vi "dvl sim (SubVI).vi"(0 "IC_Water_depth":dbl=50.0, 1 "a2":dbl, 2 "b2":dbl, 5 "a1":dbl=-0.1, 9 "b1":dbl=0.2, 13 "eta":dbl[](array[numeric])) -> (3 "f_xy":dbl, 4 "dvl_1":dbl, 6 "dvl_2":dbl, 8 "alt":dbl, 10 "dvl_3":dbl, 14 "DVL_alts":dbl[](array[numeric]), 15 "dvl_4":dbl)   [LabVIEW 2014]
uses:
  <vilib>/imath/engines/lvmath2/RunTimeEngine/IndexRead/NIMS V(S).vi
  <instcachedir>/0/NIMS V(S)_0488751826AF41519A22953C041130DC.lvgen/NIMS V(S)_0488751826AF41519A22953C041130DC_000.vi
  <vilib>/imathl/engines/lvmath/Functions/Error Handling/Create Error.vi
  <vilib>/imath/engines/lvmath2/RunTimeEngine/ArithmeticOperatorToken/NIMS_ArithmeticOperator_multmx(M,CV)-internal.vi
  <instcachedir>/0/NIMS_ArithmeticOperator_multmx(M,CV)-internal_25C7CE5937BA4322B5BE2717374345EA.lvgen/NIMS_ArithmeticOperator_multmx(M,CV)-internal_25C7CE5937BA4322B5BE2717374345EA_001.vi
  <vilib>/imath/engines/lvmath2/RunTimeEngine/RangeToken/NIMS_Range_R2 - Integer.vi
  <instcachedir>/0/NIMS_Range_R2 - Integer_2D1304BAF97744E0A293025746CBADFC.lvgen/NIMS_Range_R2 - Integer_2D1304BAF97744E0A293025746CBADFC_000.vi
  <vilib>/imath/engines/lvmath2/RunTimeEngine/CommandStatement/MC_CommandStatement_break.vi
  <vilib>/imath/engines/lvmath2/RunTimeEngine/ErrorHandling/NIMS_Create Error From Enums.vi
  <instcachedir>/0/NIMS V(S)_0488751826AF41519A22953C041130DC.lvgen/NIMS V(S)_0488751826AF41519A22953C041130DC_008.vi
  <vilib>/imath/engines/lvmath2/RunTimeEngine/IndexReplace/NIMS V(S)=S.vi
  <instcachedir>/0/NIMS V(S)=S_2D52C4EC15D8415E870AEE69FB516CCA.lvgen/NIMS V(S)=S_2D52C4EC15D8415E870AEE69FB516CCA_001.vi
  <instcachedir>/0/NIMS V(S)_0488751826AF41519A22953C041130DC.lvgen/NIMS V(S)_0488751826AF41519A22953C041130DC_006.vi
  <vilib>/imath/engines/lvmath2/RunTimeEngine/NodeEndStatement/NIMS_NodeEndStatement_Output.vi
  <instcachedir>/0/NIMS_NodeEndStatement_Output_53EC0D466D134D7ABD903AC30B43404B.lvgen/NIMS_NodeEndStatement_Output_53EC0D466D134D7ABD903AC30B43404B_001.vi
  <vilib>/imath/engines/lvmath2/RunTimeEngine/ErrorHandling/NIMS_Finalize Error.vi
panel:
  in  "dvl_do":i8[](array[numeric])=[1, 1, 1, 1]
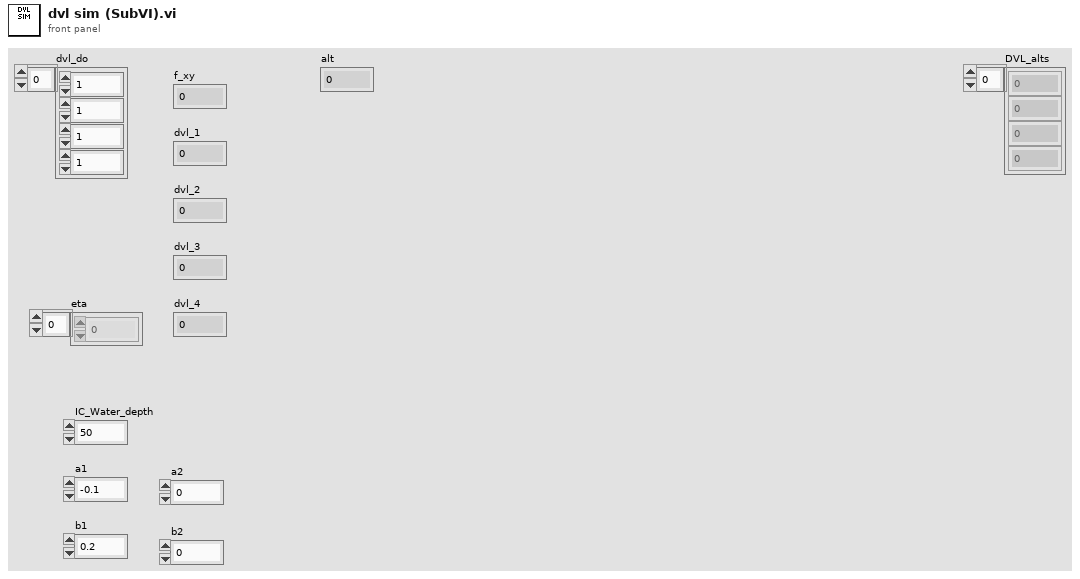
[diagram p1: front panel]
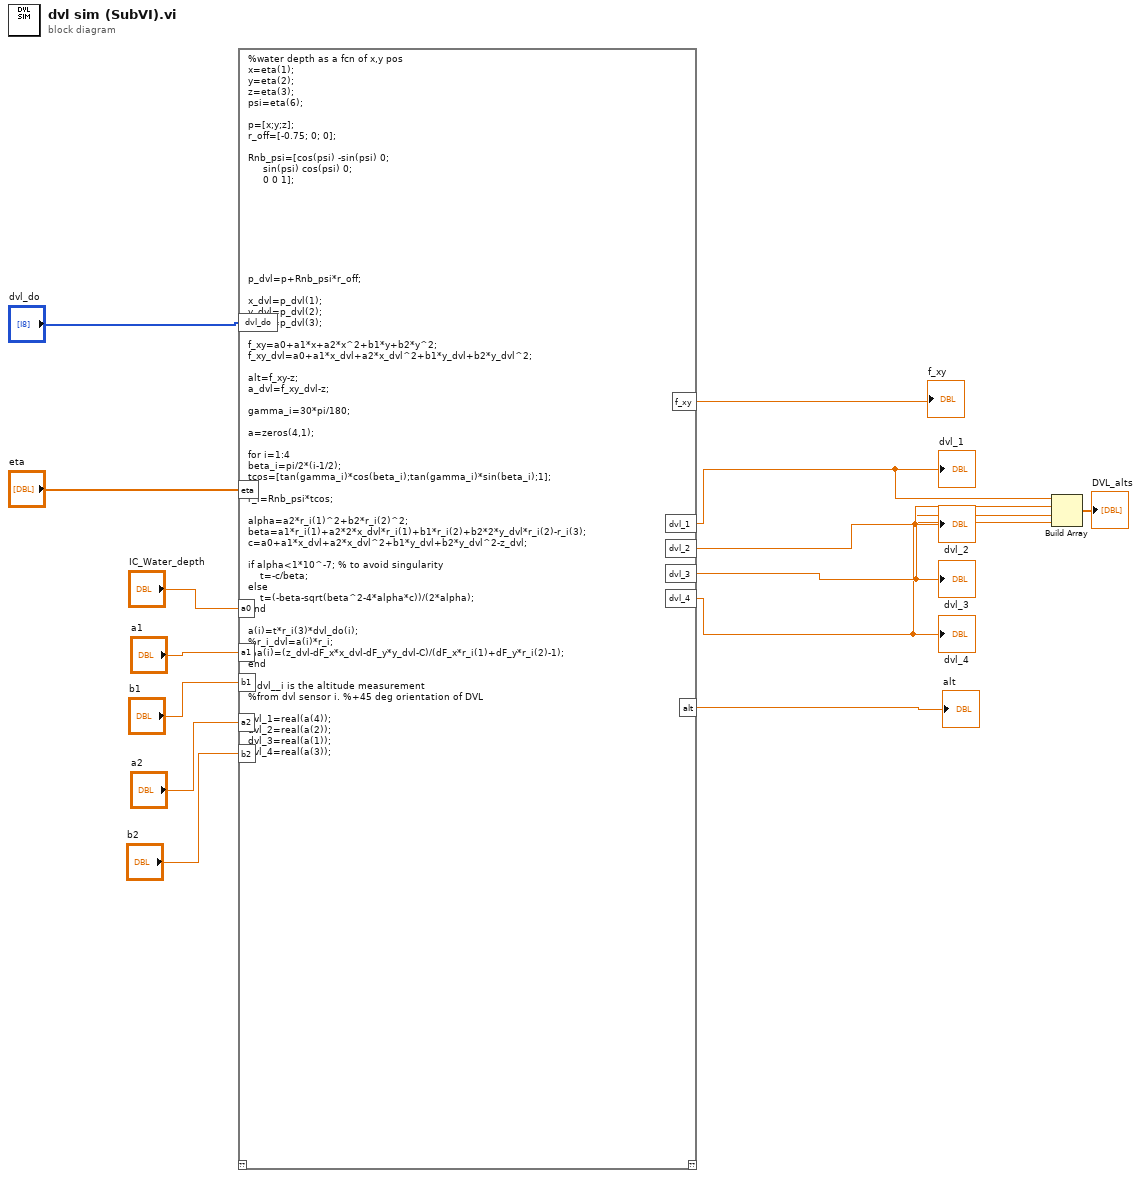
[diagram p0: block diagram]
diagram:
  n1 = mathscript code="%water depth as a fcn of x,y pos\nx=eta(1);\ny=eta(2);\nz=eta(3);\npsi=eta(6);\n\np=[x;y;z];\nr_off=[-0.75; 0; 0];\n\nRnb_psi=[cos(psi) -sin(psi) 0;\n     sin(psi) cos(psi) 0;\n     0 0 1];\n\n\n\n\n\n\n\n\np_dvl=p+Rnb_psi*r_off;\n\nx_dvl=p_dvl(1);\ny_dvl=p_dvl(2);\nz_dvl=p_dvl(3);\n\nf_xy=a0+a1*x+a2*x^2+b1*y+b2*y^2;\nf_xy_dvl=a0+a1*x_dvl+a2*x_dvl^2+b1*y_dvl+b2*y_dvl^2;\n\nalt=f_xy-z;\na_dvl=f_xy_dvl-z;\n\ngamma_i=30*pi/180;\n\na=zeros(4,1);\n\nfor i=1:4\nbeta_i=pi/2*(i-1/2);\ntcos=[tan(gamma_i)*cos(beta_i);tan(gamma_i)*sin(beta_i);1];\n\nr_i=Rnb_psi*tcos;\n\nalpha=a2*r_i(1)^2+b2*r_i(2)^2;\nbeta=a1*r_i(1)+a2*2*x_dvl*r_i(1)+b1*r_i(2)+b2*2*y_dvl*r_i(2)-r_i(3);\nc=a0+a1*x_dvl+a2*x_dvl^2+b1*y_dvl+b2*y_dvl^2-z_dvl;\n\nif alpha<1*10^-7; % to avoid singularity\n    t=-c/beta;\nelse\n    t=(-beta-sqrt(beta^2-4*alpha*c))/(2*alpha);\nend\n\na(i)=t*r_i(3)*dvl_do(i);\n%r_i_dvl=a(i)*r_i;\n%a(i)=(z_dvl-dF_x*x_dvl-dF_y*y_dvl-C)/(dF_x*r_i(1)+dF_y*r_i(2)-1);\nend\n\n%dvl__i is the altitude measurement\n%from dvl sensor i. %+45 deg orientation of DVL\n\ndvl_1=real(a(4));\ndvl_2=real(a(2));\ndvl_3=real(a(1));\ndvl_4=real(a(3));"("eta"="eta", "a0"="IC_Water_depth", "a1"="a1", "b1"="b1", "a2"="a2", "b2"="b2", "dvl_do"="dvl_do") -> ("f_xy"=→"f_xy":dbl, "dvl_1"=w5:dbl, "dvl_2"=w4:dbl, "dvl_3"=w3:dbl, "dvl_4"=w2:dbl, "alt"=→"alt":dbl)  [unwired: 1 in, 1 out]
  "dvl_4" <- w2
  "dvl_3" <- w3
  "dvl_2" <- w4
  "dvl_1" <- w5
  n2 = Build Array(w5, w4, w3, w2) -> (→"DVL_alts":dbl[])
